vi "transferPrivate.vi"(8 "error in (no error)":errorcluster, 10 "TransferFrom in":refnum<class "xceNode.lvclass">, 11 "TransferTo in":refnum<class "xceNode.lvclass">) -> (0 "error out":errorcluster, 2 "TransferFrom out":refnum<class "xceNode.lvclass">, 3 "TransferTo out":refnum<class "xceNode.lvclass">)   [LabVIEW 2013, in "xceNode.lvclass"]
doc: "Transfers the private data 'treeTag' to another node."
uses:
  xceNode.lvclass
  xceNode.lvclass/xceNode.ctl
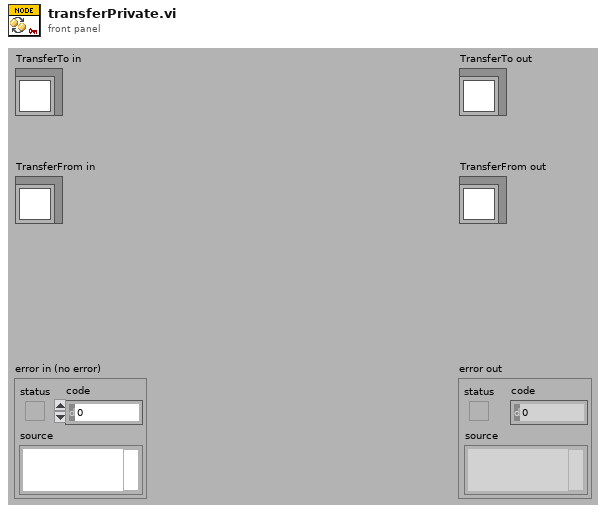
[diagram p1: front panel]
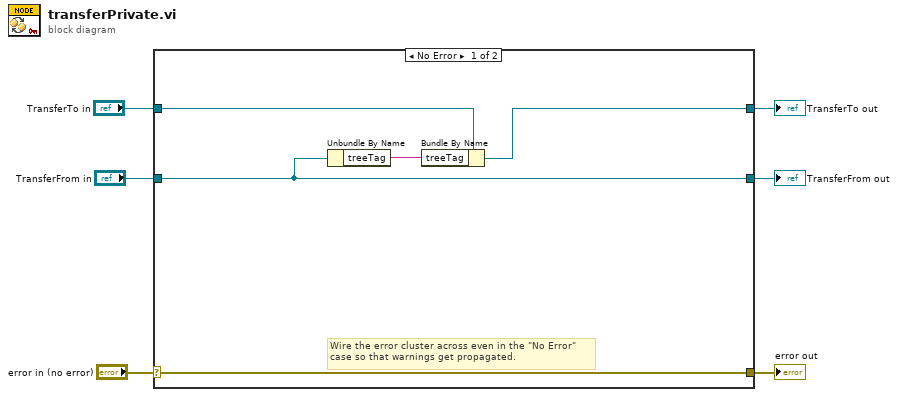
[diagram p0: block diagram]
diagram:
  n1 = case shown="No Error" "error in (no error)" {
    selector: "error in (no error)" -> [w11 w14]
    tunnel: [w11 w14] -> w5
    tunnel: [w7 w13] -> w3
    tunnel: "TransferTo in" -> [w8 w13]
    tunnel: "TransferFrom in" -> [w10 w12]
    tunnel: [w10 w12] -> w1
    frame No Error {
      # "Wire the error cluster across even in the \"No Error\"\ncase so that warnings get propagated."
      n2 = Unbundle By Name(w10) -> ("treeTag"=w9:string)
      n3 = Bundle By Name(cluster=w8, "treeTag"=w9) -> (w7:refnum<class "xceNode.lvclass">)
    }
    frame Error {
    }
  }
  "error out" <- w5
  "TransferTo out" <- w3
  "TransferFrom out" <- w1
